vi "RT Driver VI.vi"(6 "Device Clock":string, 9 "Device Inputs FIFO":refnum<k33>, 10 "Device Outputs FIFO":refnum<k33>, 11 "Device Reference":T1 format="%.0x") -> ()   [LabVIEW 2020, in "Waveform Analog Output Engine.lvlib"]
uses:
  Waveform Analog Output Engine.lvlib
  <vilib>/NI VeriStand/Custom Device API/Custom Device Item Ref.ctl
  <vilib>/NI VeriStand/Custom Device API/Custom Device Channel Type.ctl
  <vilib>/Platform/TimedLoop/XDataNode/timing_clust.ctl
  <vilib>/Platform/TimedLoop/XDataNode/nitl_modes.ctl
  <vilib>/Platform/TimedLoop/XDataNode/wakeup.ctl
  <vilib>/NI VeriStand/Custom Device API/Message Response (String).ctl
  <vilib>/NI VeriStand/Custom Device API/Message Response (Byte Array).ctl
  <vilib>/DAQmx/write.llb/DAQmx Write (Analog 1D Wfm NChan NSamp).vi
  <vilib>/DAQmx/miscellaneous.llb/DAQmx Fill In Error Info.vi
  <vilib>/platform/TimedLoop/XDataNode/XDataNode.xnode
  <vilib>/NI VeriStand/Custom Device API/Custom Device API.lvlib
  <vilib>/NI VeriStand/Custom Device Tools/Custom Device Utility Library/Custom Device Utility Library.lvlib
  <resource>/objmgr/daqmx.rc
  <vilib>/Platform/TimedLoop/XDataNode/XDNodeRunTimeDep.lvlib
panel:
  out "Number of Underflow Occurred":i32
  out "L2 Output Buffer Usage":i32
  out "Actual Update Interval_Data Loop":dbl
  out "DAQ Error Code":i32
  out "Actual Update Interval_DAQ Loop":dbl
  out "Actual Sample Rate":dbl
  in  "Initialization Status Notifier":refnum<notifier>
  in  "Status Notifier":refnum<notifier>
  # "Custom Device Template\nv1.0"
  # "Use this template as a starting point for creating a custom device code module. The input controls shown here are specially named controls that the system will use to provide the device loop with data. The controls are not required for the device loop to run. For instance, if the device doesn't produce any output data, then you don't need the Device Outputs FIFO control. If you do use these controls, however, they need to have these exact names to be functional."
  # "status chs"
  # "The optional status notifier element is used to notify the RT engine of the last state of the custom device, and to indicate the device has completed execution. If this control is not used, a default No Error value is returned to the system when the device finishes execution.\n\nNote: This error state is not checked until the system shuts down. Use an output status channel to send more immediate status values to the system."
  # "This optional input can be used to send the VeriStand Engine the final status of the custom device initalization process. If this control exists on the custom device front panel, the VeriStand Engine will wait for a status update before starting up. If the custom device reports an error, that will abort the execution of the current configuration in the VeriStand Engine.\n\nThis control can be deleted if the custom device does not need to send the initialization status update."
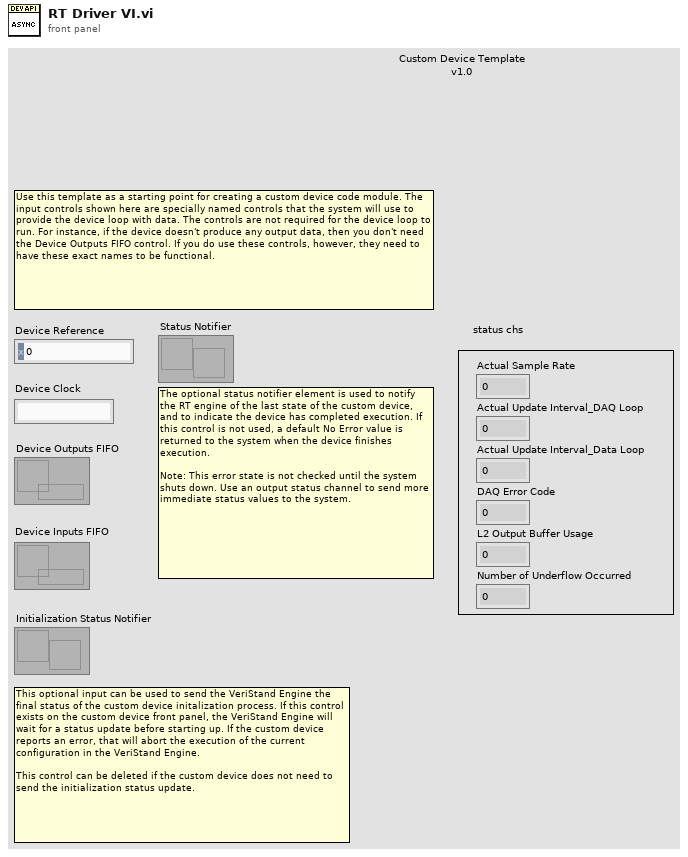
[diagram p1: front panel]
types:
  T1 = typedef "Custom Device API.lvlib/Custom Device Item Ref.ctl" = u64
  T2 = typedef "Custom Device API.lvlib/Custom Device Channel Type.ctl" = enum16{"Input", "Output"}
  T3 = typedef "Custom Device API.lvlib/Custom Device Engine Event Ref.ctl" = refnum<event-registration>
  T4 = typedef "Custom Device API.lvlib/Custom Device Timed Loop Priority.ctl" = enum32{"Low", "Medium", "High"}
  T5 = typedef "XDNodeRunTimeDep.lvlib/timing_clust.ctl" = cluster{"Expected End [f-1]":u64, "Actual End [f-1]":u64, "Finished Late? [f-1]":bool, "Expected End [i-1]":u64, "Actual End [i-1]":u64, "Finished Late? [i-1]":bool, "Expected Start [i]":u64, "Actual Start [i]":u64, "Expected Start [f]":u64, "Actual Start [f]":u64, "Source Name":string, "Structure Name":string, "Period":i64, "Deadline":i64, "Offset":i64, "Start":i64, "Priority":i32, "Timeout":i32, "Mode":T6, "Wakeup Reason":T7, "Error":errorcluster, "Source Type":string, "Secondary Source Type":string, "Global End Time":u64, "Global Start Time":u64, "Frame Duration":u64, "Iteration Duration":u64, "Assigned CPU":i32, "I/O Scan Engine Mode":u32}
  T6 = typedef "XDNodeRunTimeDep.lvlib/nitl_modes.ctl" = enum32{"No Change", "Process missed periods, maintain original phase", "Discard missed periods, maintain original phase", "Process missed periods, ignore original phase", "Discard missed periods, ignore original phase"}
  T7 = typedef "XDNodeRunTimeDep.lvlib/wakeup.ctl" = enum32{"Normal", "Aborted", "Asynchronous wakeup", "Timing source error", "Timed loop error", "Timeout"}
  T8 = typedef "Custom Device API.lvlib/Message Response (String).ctl" = cluster{"Response":string, "Error":errorcluster}
  T9 = typedef "Custom Device API.lvlib/Message Response (Byte Array).ctl" = cluster{"Response":u8[], "Error":errorcluster}
  T10 = typedef "Waveform Analog Output Engine.lvlib/DAQ Config Data.ctl" = cluster{"DAQPhysicalChannel(s)":string, "SampleRate":dbl, "MaxV":dbl, "MinV":dbl, "#Samples":dbl, "DataLoopInterval(ms)":u32, "StartDelay(ms)":dbl, "#L1OutputBuffers":dbl, "#Channels":i32, "ActualSampleRate(Hz)":dbl, "DAQTaskRef":refnum<k21>, "Latency":dbl}
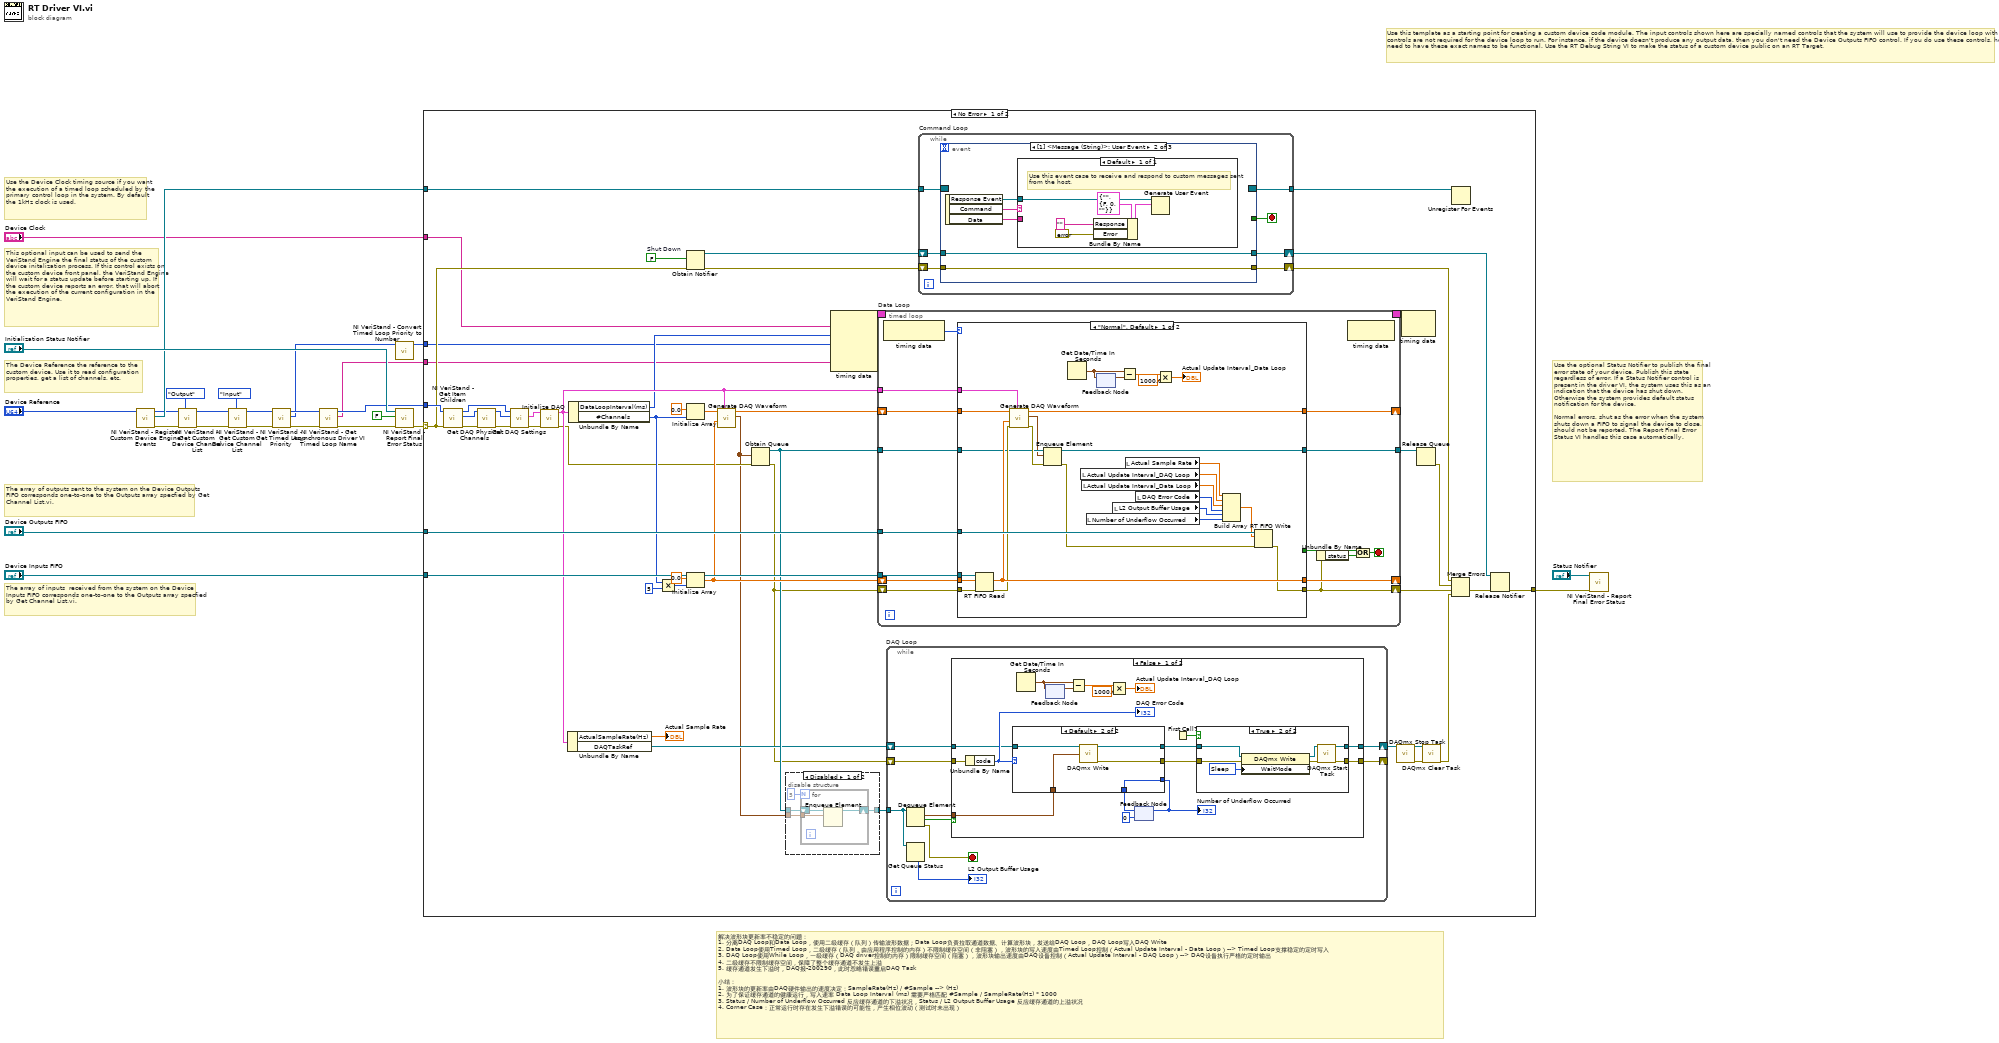
[diagram p0: block diagram]
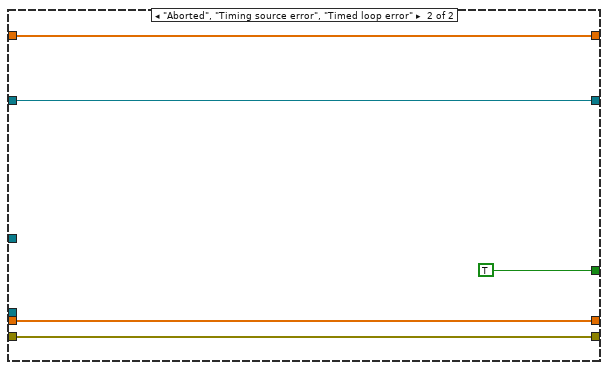
[diagram p3: hidden frame]
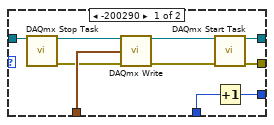
[diagram p4: hidden frame]
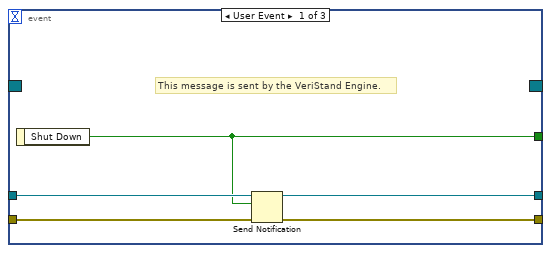
[diagram p7: hidden frame]
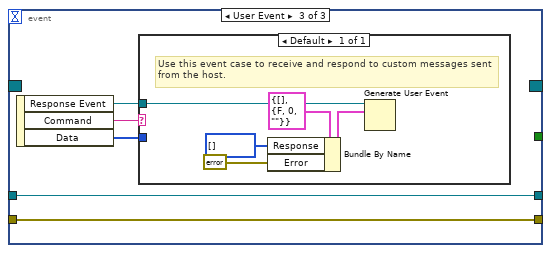
[diagram p8: hidden frame]
diagram:
  # "解决波形块更新率不稳定的问题：\n1. 分离DAQ Loop和Data Loop，使用二级缓存（队列）传输波形数据；Data Loop负责拉取通道数据、计算波形块，发送给DAQ Loop，DAQ Loop写入DAQ Write\n2. Data Loop使用Timed Loop，二级缓存（队列，由应用程序控制的内存）不限制缓存空间（非阻塞），波形块的写入速度由Timed Loop控制（Actual Update Interval - Data Loop）--> Timed Loop支撑稳定的定时写入\n3. DAQ Loop使用While Loop，一级缓存（DAQ driver控制的内存）限制缓存空间（阻塞），波形块输出速度由DAQ设备控制（Actual Update Interval - DAQ Loop）--> DAQ设备执行严格的定时输出\n4. 二级缓存不限制缓存空间，保障了整个缓存通道不发生上溢\n5. 缓存通道发生下溢时，DAQ报-200290，此时忽略错误重启DAQ Task\n\n小结：\n1. 波形块的更新率由DAQ硬件输出的速度决定：SampleRate(Hz) / #Sample --> (Hz)\n2. 为了保证缓存通道的健康运行，写入速率 Data Loop Interval (ms) 需要严格匹配 #Sample / SampleRate(Hz) * 1000\n3. Status / Number of Underflow Occurred 反应缓存通道的下溢状况，Status / L2 Output Buffer Usage 反应缓存通道的上溢状况\n4. Corner Case：正常运行时存在发生下溢错误的可能性，产生相位波动（测试时未出现）"
  # "This optional input can be used to send the VeriStand Engine the final status of the custom device initalization process. If this control exists on the custom device front panel, the VeriStand Engine will wait for a status update before starting up. If the custom device reports an error, that will abort the execution of the current configuration in the VeriStand Engine."
  # "The array of inputs  received from the system on the Device Inputs FIFO corresponds one-to-one to the Outputs array specfied by Get Channel List.vi."
  # "Use the optional Status Notifier to publish the final error state of your device. Publish this state regardless of error. If a Status Notifier control is present in the driver VI, the system uses this as an indication that the device has shut down. Otherwise the system provides default status notification for the device.\n\nNormal errors, shut as the error when the system shuts down a FIFO to signal the device to close, should not be reported. The Report Final Error Status VI handles this case automatically."
  # "The array of outputs sent to the system on the Device Outputs FIFO corresponds one-to-one to the Outputs array specfied by Get Channel List.vi."
  # "The Device Reference the reference to the custom device. Use it to read configuration properties, get a list of channels, etc."
  # "Use the Device Clock timing source if you want the execution of a timed loop scheduled by the primary control loop in the system. By default the 1kHz clock is used."
  # "Use this template as a starting point for creating a custom device code module. The input controls shown here are specially named controls that the system will use to provide the device loop with data. The controls are not required for the device loop to run. For instance, if the device doesn't produce any output data, then you don't need the Device Outputs FIFO control. If you do use these controls, however, they need to have these exact names to be functional. Use the RT Debug String VI to make the status of a custom device public on an RT Target."
  n1 = call <vilib>:"NI VeriStand - Register Custom Device Engine Events.vi"("Device Ref in"="Device Reference") -> ("error out"=w25:errorcluster, "Custom Device Engine Event Ref"=w16:T3, "Device Ref out"=w14:T1)  [unwired: 8 in]
  n2 = call <vilib>:"NI VeriStand - Get Custom Device Channel List.vi"("Channel Type"=Custom_Device_Channel_Type."Output", "error in (no error)"=w25, "Device Ref in"=w14) -> ("error out"=w19:errorcluster, "Device Ref out"=w20:T1)  [unwired: 7 out]
  n3 = call <vilib>:"NI VeriStand - Get Custom Device Channel List.vi"("Channel Type"=Custom_Device_Channel_Type."Input", "error in (no error)"=w19, "Device Ref in"=w20) -> ("error out"=w3:errorcluster, "Device Ref out"=w12:T1)  [unwired: 7 out]
  n4 = call <vilib>:"NI VeriStand - Get Timed Loop Priority.vi"("error in (no error)"=w3, "Device Ref in"=w12) -> ("error out"=w2:errorcluster, "Priority"=w7:T4, "Device Ref out"=w9:T1)  [unwired: 7 in]
  n5 = call <vilib>:"NI VeriStand - Get Asynchronous Driver VI Timed Loop Name.vi"("error in (no error)"=w2, "Device Ref in"=w9) -> ("error out"=w1:errorcluster, "Device Timed Loop Name"=w4:string, "Device Ref out"=w5:T1)  [unwired: 7 in]
  n6 = call <vilib>:"NI VeriStand - Convert Timed Loop Priority to Number.vi"("Priority"=w7) -> ("Numeric Priority"=w6:i32)  [unwired: 10 in]
  n7 = call <vilib>:"NI VeriStand - Report Final Error Status.vi"("error in (no error)"=w1, "Filter FIFO & Shutdown Errors (T)"=FALSE ("Filter FIFO Errors (T)"), "Status Notifier"="Initialization Status Notifier") -> ("error out"=w10:errorcluster)  [unwired: 8 out]
  n8 = case shown="No Error" w10 {
    selector: w10 -> [w52 w224]
    tunnel: "Device Outputs FIFO" -> [w73 _]
    tunnel: "Device Inputs FIFO" -> [w72 _]
    tunnel: w16 -> [w70 _]
    tunnel: [w68 w224] -> w15
    tunnel: w5 -> [w61 _]
    tunnel: "Device Clock" -> [w33 _]
    tunnel: w6 -> [w32 _]
    tunnel: w4 -> [w31 _]
    frame No Error {
      w69 = FALSE  # Shut Down
      n9 = call <vilib>:"NI VeriStand - Get Item Children.vi"("error in (no error)"=w52, "Item Ref in"=w61) -> ("error out"=w63:errorcluster, "Child Refs"=w58:T1[], "Item Ref out"=w59:T1)  [unwired: 6 in, 1 out]
      n10 = call "Get DAQ Physical Channels.vi"("error in (no error)"=w63, "DAQ Channel Section Refs"=w58) -> ("error out"=w62:errorcluster, "Physical Channels"=w60:i32[])  [unwired: 8 in]
      n11 = call "Get DAQ Settings.vi"("error in (no error)"=w62, "Physical Chan Array"=w60, "Device Ref in"=w59) -> ("error out"=w51:errorcluster, "DAQ Config Data"=w50:T10)  [unwired: 6 in, 1 out]
      n12 = call "Initialize DAQ.vi"("error in (no error)"=w51, "DAQ Config Data In"=w50) -> ("error out"=w43:errorcluster, "DAQ Config Data Out"=w44:T10)  [unwired: 8 in]
      n13 = Unbundle By Name(w44) -> ("ActualSampleRate(Hz)"=→"Actual Sample Rate":dbl, "DAQTaskRef"=w39:refnum<k21>)
      n14 = Unbundle By Name(w44) -> ("DataLoopInterval(ms)"=w34:u32, "#Channels"=w54:i32)
      n15 = Multiply(x=w54, y=5) -> (x*y=w56:i32)
      n16 = Obtain Notifier(notification data type=w69, error in (no error)=w52) -> (notifier out=w66:refnum<notifier>, error out=w74:errorcluster)  [unwired: 2 in, 1 out]
      n17 = Initialize Array(0.0 ("element"), w54) -> (w49:dbl[])
      n18 = Initialize Array(0.0 ("element"), w56) -> (w47:dbl[])
      n19 = call "Generate DAQ Waveform.vi"("DAQ Config Data"=w44, "Channel Data"=w47, "Phase Array In"=w49) -> ("Waveform Array"=w37:waveform(dbl)[], "Phase Array Out out"=w48:dbl[])  [unwired: 6 in, 1 out]
      n20 = Obtain Queue(element data type=w37, error in (no error)=w43) -> (queue out=w42:refnum<queue>, error out=w38:errorcluster)  [unwired: 3 in, 1 out]
      n21 = disable-structure shown="Disabled" {
        disable-tunnel: [w78 w82] -> w46
        disable-tunnel: w42 -> [w76 w82]
        disable-tunnel: w37 -> [w75 _]
        frame Disabled {
          n22 = for {
            N: 5 -> [_]
            tunnel: w75 -> [w79]
            shift-right: [w80] -> w78
            shift-left: w76 -> [w81]
            n23 = Enqueue Element(queue=w81, element=w79) -> (queue out=w80:refnum<queue>)  [unwired: 2 in, 2 out]
          }
        }
        frame Enabled {
        }
      }
      n24 = node-c288(w33, w34, w32, w31) -> (w36:T5)  [unwired: 1 in]
      n25 = timed-loop "Data Loop" {
        shift-right: [w95] -> _
        shift-left: w47 -> [w96]
        shift-right: [w92] -> w40
        shift-left: w38 -> [w97]
        tunnel: w73 -> [w94]
        tunnel: w72 -> [w93]
        shift-right: [w87] -> _
        shift-left: w48 -> [w88]
        tunnel: w44 -> [w86]
        tunnel: w42 -> [w85]
        tunnel: [w84] -> w41
        timing: w36 -> [_]
        timing-out: [_] -> w35
        stop <- w89 stop-if-true
        n26 = node-c288() -> (w83:T7)  [unwired: 1 in]
        n27 = case shown="\"Normal\", Default" w83 {
          tunnel: w97 -> [w119 w131]
          tunnel: w96 -> [w123 w132]
          tunnel: [w122 w132] -> w95
          tunnel: w94 -> [w127 _]
          tunnel: w93 -> [w126 _]
          tunnel: [w121 w131] -> w92
          tunnel: [_ TRUE] -> w90
          tunnel: w88 -> [w124 w129]
          tunnel: [w125 w129] -> w87
          tunnel: w86 -> [w120 _]
          tunnel: w85 -> [w116 w128]
          tunnel: [w113 w128] -> w84
          frame "Normal", Default {
            n28 = RT FIFO Read(0:w126, 1:w123, 3:w119) -> (9:w122:dbl[], 11:w118:errorcluster)  [unwired: 4 out]
            n29 = call "Generate DAQ Waveform.vi"("DAQ Config Data"=w120, "error in (no error)"=w118, "Channel Data"=w122, "Phase Array In"=w124) -> ("error out"=w117:errorcluster, "Waveform Array"=w114:waveform(dbl)[], "Phase Array Out out"=w125:dbl[])  [unwired: 5 in]
            n30 = Enqueue Element(queue=w116, element=w114, error in (no error)=w117) -> (queue out=w113:refnum<queue>, error out=w115:errorcluster)  [unwired: 1 in, 1 out]
            n31 = Get Date/Time In Seconds() -> (seconds since 1Jan1904=w109:timestamp)
            n32 = local read "Actual Update Interval_DAQ Loop"() -> (w103:dbl)
            n33 = local read "Actual Update Interval_Data Loop"() -> (w104:dbl)
            n34 = local read "Number of Underflow Occurred"() -> (w107:i32)
            n35 = feedback #1() -> (w110:timestamp)  [unwired: 1 in]
            n36 = feedback-in #1(w109) -> ()
            n37 = local read "L2 Output Buffer Usage"() -> (w101:i32)
            n38 = Subtract(x=w109, y=w110) -> (x-y=w111:dbl)
            n39 = local read "Actual Sample Rate"() -> (w106:dbl)
            n40 = local read "DAQ Error Code"() -> (w105:i32)
            n41 = Multiply(x=w111, y=1000.0) -> (x*y=→"Actual Update Interval_Data Loop":dbl)
            n42 = Build Array(w106, w103, w104, w105, w101, w107) -> (w102:dbl[])
            n43 = RT FIFO Write(0:w127, 1:w102, 3:w115) -> (11:w121:errorcluster)  [unwired: 1 in, 4 out]
          }
          frame "Aborted", "Timing source error", "Timed loop error" {
          }
        }
        n44 = Unbundle By Name(w92) -> ("status"=w91:bool)
        n45 = node-c288() -> ()  [unwired: 1 in, 1 out]
        n46 = Compound Arithmetic op=OR(w90, w91) -> (w89:bool)
      }
      n47 = while "DAQ Loop" {
        shift-right: [w148] -> w45
        shift-left: w39 -> [w147]
        tunnel: w46 -> [w141]
        shift-right: [w144] -> _
        shift-left: w38 -> [w143]
        stop <- w142 stop-if-true
        n48 = Dequeue Element(queue=w141) -> (element=w145:waveform(dbl)[], timed out?=w146:bool, error out=w142:errorcluster)  [unwired: 2 in, 1 out]
        n49 = Get Queue Status(queue=w141) -> (# elements in queue=→"L2 Output Buffer Usage":i32)  [unwired: 2 in, 7 out]
        n50 = case shown="False" w146 {
          tunnel: [w164 w191] -> w148
          tunnel: w147 -> [w156 w191]
          tunnel: w145 -> [w155 _]
          tunnel: [w159 w190] -> w144
          tunnel: w143 -> [w158 w190]
          frame False {
            n51 = Unbundle By Name(w158) -> ("code"=w157:i32)
            "DAQ Error Code" <- w157
            n52 = Get Date/Time In Seconds() -> (seconds since 1Jan1904=w160:timestamp)
            n53 = feedback #2() -> (w161:timestamp)  [unwired: 1 in]
            n54 = feedback-in #2(w160) -> ()
            n55 = Subtract(x=w160, y=w161) -> (x-y=w162:dbl)
            n56 = Multiply(x=w162, y=1000.0) -> (x*y=→"Actual Update Interval_DAQ Loop":dbl)
            n57 = feedback #3(0) -> (w151:i32)
            n58 = case shown="Default" w157 {
              tunnel: [w175 w178] -> w153
              tunnel: w156 -> [w174 w179]
              tunnel: w155 -> [w173 w180]
              tunnel: [w168 w177] -> w154
              tunnel: [w166 w176] -> w150
              tunnel: w151 -> [w167 w176]
              frame -200290 {
                n59 = call <vilib>:"DAQmx Stop Task.vi"("task/channels in"=w174) -> ("task out"=w172:refnum<k21>, "error out"=w171:errorcluster)  [unwired: 13 in]
                n60 = call-poly <vilib>:"DAQmx Write.vi"("task/channels in"=w172, "data"=w173, "error in"=w171) -> ("task out"=w169:refnum<k21>, "error out"=w170:errorcluster)  [unwired: 10 in, 1 out]
                n61 = call <vilib>:"DAQmx Start Task.vi"("task/channels in"=w169, "error in"=w170) -> ("task out"=w168:refnum<k21>, "error out"=w175:errorcluster)  [unwired: 12 in]
                n62 = Increment(x=w167) -> (x+1=w166:i32)
              }
              frame Default {
                n63 = call-poly <vilib>:"DAQmx Write.vi"("task/channels in"=w179, "data"=w180) -> ("task out"=w177:refnum<k21>, "error out"=w178:errorcluster)  [unwired: 11 in, 1 out]
              }
            }
            "Number of Underflow Occurred" <- w150
            n64 = feedback-in #3(w150) -> ()
            n65 = First Call?() -> (First Call?: T/F=w165:bool)
            n66 = case shown="True" w165 {
              tunnel: w154 -> [w182 w186]
              tunnel: [w182 w185] -> w164
              tunnel: w153 -> [w181 w184]
              tunnel: [w181 w183] -> w159
              frame False {
              }
              frame True {
                w187 = 12547 items=["Poll"=12524, "Yield"=12525, "Sleep"=12547] ("WaitMode")
                n67 = property class="DAQmx Write"(reference=w186, error in=w184, "WaitMode"=w187) -> (reference out=w189:refnum<k21>, error out=w188:errorcluster)
                n68 = call <vilib>:"DAQmx Start Task.vi"("task/channels in"=w189, "error in"=w188) -> ("task out"=w185:refnum<k21>, "error out"=w183:errorcluster)  [unwired: 12 in]
              }
            }
          }
          frame True {
          }
        }
      }
      n69 = while "Command Loop" {
        tunnel: w70 -> [w198]
        tunnel: [w197] -> w67
        shift-right: [w194] -> w65
        shift-left: w66 -> [w195]
        shift-right: [w192] -> w27
        shift-left: w74 -> [w193]
        stop <- w196 stop-if-true
        n70 = event shown="[1] <Message (String)>: User Event" {
          selector: w198 -> [_ _ _]
          dyn-events: [_ _ _] -> w197
          timeout: _ -> [_ _ _]
          tunnel: [w201 _ _] -> w196
          tunnel: w195 -> [w202 w206 w216]
          tunnel: [w203 w206 w216] -> w194
          tunnel: w193 -> [w200 w204 w214]
          tunnel: [w199 w204 w214] -> w192
          event User Event {
            # "This message is sent by the VeriStand Engine."
            n71 = event-data() -> ("Shut Down"=w201:bool)  [unwired: 1 in]
            n72 = Send Notification(notification=w201, notifier=w202, error in (no error)=w200) -> (notifier out=w203:refnum<notifier>, error out=w199:errorcluster)
          }
          event User Event {
            n73 = event-data() -> ("Response Event"=w205:refnum<user-event>, "Command"=w208:string, "Data"=w207:string)  [unwired: 1 in]
            n74 = case shown="Default" w208 {
              tunnel: w207 -> [_]
              tunnel: w205 -> [w213]
              frame Default {
                # "Use this event case to receive and respond to custom messages sent from the host."
                n75 = Bundle By Name(cluster=T8 {"Response"="", "Error"={"status"=FALSE, "code"=0, "source"=""}} ("event data"), "Response"="", "Error"=errorcluster {"status"=FALSE, "code"=0, "source"=""}) -> (w211:T8)
                n76 = Generate User Event(user event=w213, event data cluster=w211) -> ()  [unwired: 2 in, 2 out]
              }
            }
          }
          event User Event {
            n77 = event-data() -> ("Response Event"=w215:refnum<user-event>, "Command"=w218:string, "Data"=w217:u8[])  [unwired: 1 in]
            n78 = case shown="Default" w218 {
              tunnel: w217 -> [_]
              tunnel: w215 -> [w223]
              frame Default {
                # "Use this event case to receive and respond to custom messages sent from the host."
                n79 = Bundle By Name(cluster=T9 {"Response"=[], "Error"={"status"=FALSE, "code"=0, "source"=""}} ("event data"), "Response"=u8[] [], "Error"=errorcluster {"status"=FALSE, "code"=0, "source"=""}) -> (w220:T9)
                n80 = Generate User Event(user event=w223, event data cluster=w220) -> ()  [unwired: 2 in, 2 out]
              }
            }
          }
        }
      }
      n81 = call <vilib>:"DAQmx Stop Task.vi"("task/channels in"=w45) -> ("task out"=w53:refnum<k21>, "error out"=w29:errorcluster)  [unwired: 13 in]
      n82 = node-c288(w35) -> ()  [unwired: 1 out]
      n83 = Release Queue(queue=w41) -> (error out=w26:errorcluster)  [unwired: 2 in, 2 out]
      n84 = call <vilib>:"DAQmx Clear Task.vi"("task in"=w53, "error in"=w29) -> ("error out"=w28:errorcluster)  [unwired: 13 in]
      n85 = Merge Errors(w27, w26, w40, w28) -> (w64:errorcluster)
      n86 = Unregister For Events(event registration refnum=w67) -> ()  [unwired: 1 in, 1 out]
      n87 = Release Notifier(notifier=w65, error in (no error)=w64) -> (error out=w68:errorcluster)  [unwired: 1 in, 2 out]
    }
    frame Error {
    }
  }
  n88 = call <vilib>:"NI VeriStand - Report Final Error Status.vi"("error in (no error)"=w15, "Status Notifier"="Status Notifier") -> ()  [unwired: 1 in, 9 out]
